vi "Finalize.vi"(8 "error in":errorcluster, 11 "Plugin in":refnum<class "RPM Plugin.lvclass">) -> (0 "error out":errorcluster, 3 "Plugin out":refnum<class "RPM Plugin.lvclass">)   [LabVIEW 2020, in "RPM Plugin.lvlib" / "RPM Plugin.lvclass"]
uses:
  RPM Plugin.lvclass
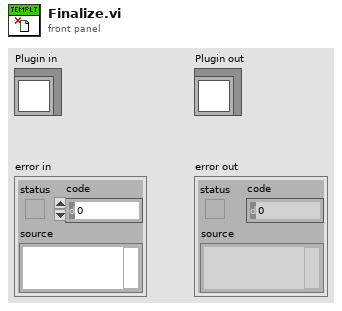
[diagram p1: front panel]
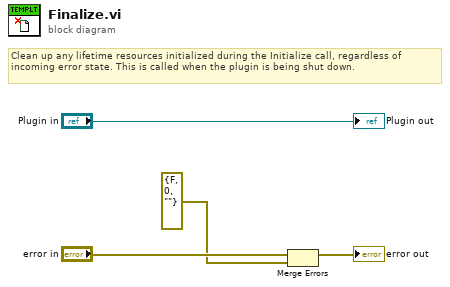
[diagram p0: block diagram]
diagram:
  # "Clean up any lifetime resources initialized during the Initialize call, regardless of incoming error state. This is called when the plugin is being shut down."
  n1 = Merge Errors("error in", errorcluster {"status"=FALSE, "code"=0, "source"=""} ("error in")) -> (→"error out":errorcluster)
  "Plugin out" <- "Plugin in"
